vi "QueueSolenAdv.vi"(0 "Statue_IN":refnum<queue>, 5 "PlatNum_IN":refnum<queue>, 7 "Statue_Value":i32, 9 "PlatNum_Value":i32, 11 "错误输入（无错误）":errorcluster) -> (4 "Statue_OUT":refnum<queue>, 6 "PlatNum_OUT":refnum<queue>, 15 "错误输出":errorcluster)   [LabVIEW 2011]
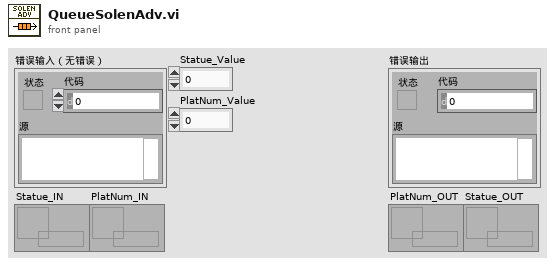
[diagram p1: front panel]
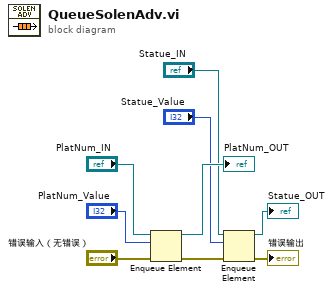
[diagram p0: block diagram]
diagram:
  n1 = Enqueue Element(queue="PlatNum_IN", element="PlatNum_Value", error in (no error)="错误输入（无错误）") -> (queue out=→"PlatNum_OUT":refnum<queue>, error out=w9:errorcluster)  [unwired: 1 in, 1 out]
  n2 = Enqueue Element(queue="Statue_IN", element="Statue_Value", error in (no error)=w9) -> (queue out=→"Statue_OUT":refnum<queue>, error out=→"错误输出":errorcluster)  [unwired: 1 in, 1 out]
